vi "Tool Common analog Variables.vi"(11 "error in (no error)":errorcluster, 13 "Tool folder name":string) -> (8 "Common Variables Fixed":T7[](array[typedef]) {"Default Scaling"."Offset" format="%.5f"; "Default Scaling"."Gain" format="%.5f"}, 10 "Common variables User settigns":T1[](array[typedef]) {"Scaling"."Offset" format="%.5f"; "Scaling"."Gain" format="%.5f"; "Limits and responces"."Limits"."H" format="%.3f"; "Limits and responces"."Limits"."L" format="%.3f"; "Limits and responces"."Limits"."HH" format="%.3f"; "Limits and responces"."Limits"."LL" format="%.3f"; "Limits and responces"."HH"."Action" items=["No Action", "Turn Off HV"]; "Limits and responces"."H"."Action" items=["No Action", "Turn Off HV"]; "Limits and responces"."L"."Action" items=["No Action", "Turn Off HV"]; "Limits and responces"."LL"."Action" items=["No Action", "Turn Off HV"]; "Limits and responces"."Technical Error(NA)"."Action" items=["No Action", "Turn Off HV"]}, 15 "error out":errorcluster)   [LabVIEW 2011]
uses:
  Measurments Handling/Fixed Analog Channel Definition.ctl
  Measurments Handling/Update frequensies.ctl
  Measurments Handling/Channel catagory Enum.ctl
  Measurments Handling/Scaling.ctl
  Measurments Handling/User Setting Analog Channel Bg.ctl
  Measurments Handling/Alarm Setup Analog.ctl
  Measurments Handling/Alarm Responce.ctl
  Measurments Handling/Action List.ctl
  Measurments Handling/Limits.ctl
  Tool/Stroker/High level/Variable List Stroker Analog.ctl
  <vilib>/Utility/VariantDataType/GetNumericInfo.vi
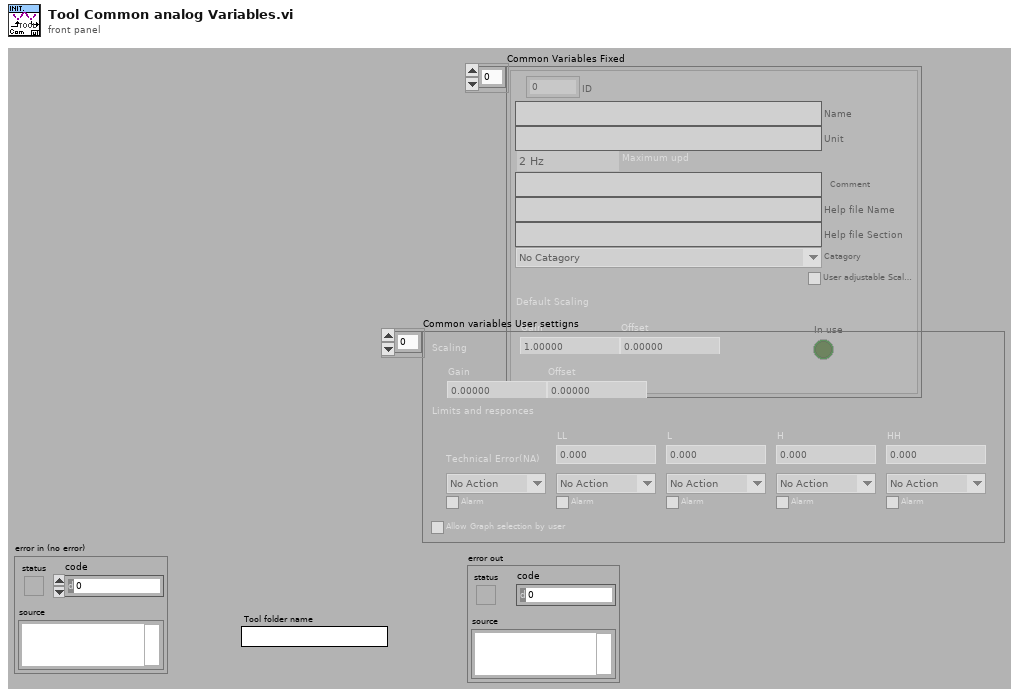
[diagram p1: front panel]
types:
  T1 = typedef "User Setting Analog Channel Bg.ctl" = cluster{"Scaling":T2, "Limits and responces":T3, "Allow Graph selection by user":bool}
  T2 = typedef "Scaling.ctl" = cluster{"Gain":dbl, "Offset":dbl}
  T3 = typedef "Alarm Setup Analog.ctl" = cluster{"Technical Error(NA)":T4, "LL":T4, "L":T4, "H":T4, "HH":T4, "Limits":T6}
  T4 = typedef "Alarm Responce.ctl" = cluster{"Action":T5, "Alarm":bool}
  T5 = typedef "Action List.ctl" = u16
  T6 = typedef "Limits.ctl" = cluster{"LL":dbl, "L":dbl, "H":dbl, "HH":dbl}
  T7 = typedef "Fixed Analog Channel Definition.ctl" = cluster{"ID":u16, "Name":string, "Unit":string, "Maximum upd":T8, "Comment":string, "Help file Name":string, "Help file Section ":string, "Catagory":T9, "User adjustable Scaling":bool, "Default Scaling":T2, "In use":bool}
  T8 = typedef "Update frequensies.ctl" = enum16{"2 Hz", "1 Hz", "0.1 Hz"}
  T9 = typedef "Channel catagory Enum.ctl" = enum16{"No Catagory", "Power", "Temperature", "Pressure"}
  T10 = typedef "Variable List Stroker Analog.ctl" = enum16{"Tool max Temperature", "Solenoid Temp", "Tool supply Voltage", "Tool (Controller) Current", "Tool Acceleration X", "Tool Acceleration Y", "Tool Acceleration Z", "Controller Temp", "Tool Acceleration Sum", "Tool Inclination", "Tool Rotation", "Tool Stroke Extension", "Tool GP Sensor 1", "Tool GP Sensor 2", "Tool (Pressure 1) Temp", "Tool Pressure 1", "Tool (Pressure 2) Temp", "Tool Pressure 2", "Do not use (SIF)", "Do not use (SOF)", "Stroke Force", "PSU Temp", "Head Voltage", "PSU Main Voltage out", "PSU Main Current out", "Tension Sub1 Temp", "Tool Tension Sub1", "Tension Sub2 Temp", "Tool Tension Sub2"}
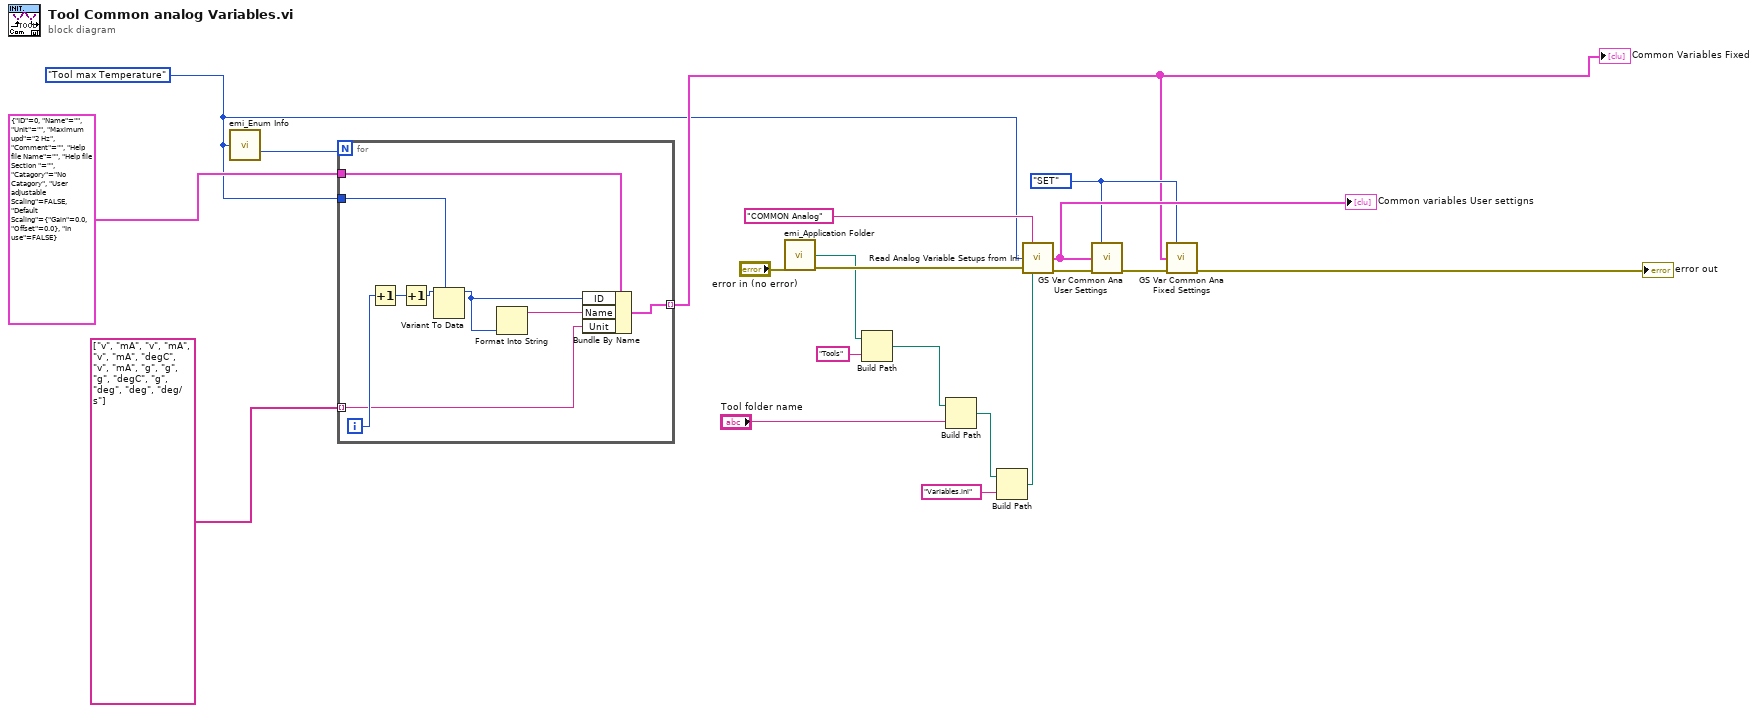
[diagram p0: block diagram]
diagram:
  w7 = Variable_List_Stroker_Analog."Tool max Temperature" ("Action")
  w15 = enum16{"GET", "SET"}."SET" ("Action(GET)")
  n1 = call "emi_Enum Info.vi"("Enum"=w7) -> ("Numb Elements"=w6:i32)  [unwired: 11 in, 3 out]
  n2 = for {
    N: w6 -> [_]
    tunnel: w7 -> [w27]
    tunnel: T7 {"ID"=0, "Name"="", "Unit"="", "Maximum upd"=enum."2 Hz", "Comment"="", "Help file Name"="", "Help file Section "="", "Catagory"=enum."No Catagory", "User adjustable Scaling"=FALSE, "Default Scaling"={"Gain"=0.0, "Offset"=0.0}, "In use"=FALSE} ("Variable Defenition") -> [w22]
    tunnel: [w23] -> w8 mode=indexing
    tunnel: string[] ["v", "mA", "v", "mA", "v", "mA", "degC", "v", "mA", "g", "g", "g", "degC", "g", "deg", "deg", "deg/s"] -> [w21] mode=indexing
    i -> [w29]
    n3 = Increment(x=w29) -> (x+1=w28:i32)
    n4 = Increment(x=w28) -> (x+1=w26:i32)
    n5 = Variant To Data(type=w27, Variant=w26) -> (data=w24:T10)  [unwired: 1 in, 1 out]
    n6 = Format Into String(w24) -> (resulting string=w25:string)  [unwired: 3 in, 1 out]
    n7 = Bundle By Name(cluster=w22, "ID"=w24, "Name"=w25, "Unit"=w21) -> (w23:T7)
  }
  "Common Variables Fixed" <- w8
  n8 = call "emi_Application Folder.vi"("error in (no error)"="error in (no error)") -> ("Dir"=w2:path, "error out"=w11:errorcluster)  [unwired: 13 in]
  n9 = Build Path(base path=w2, name or relative path="Tools") -> (appended path=w1:path)
  n10 = Build Path(base path=w1, name or relative path="Tool folder name") -> (appended path=w4:path)
  n11 = Build Path(base path=w4, name or relative path="Variables.ini") -> (appended path=w10:path)
  n12 = call "Read Analog Variable Setups from Ini.vi"("error in (no error)"=w11, "Path"=w10, "Enum with Variable List"=w7, "Section(\"Default\")"="COMMON Analog" ("Section(\"Default\")")) -> ("error out"=w19:errorcluster, "Analog User settigns"=w18:T1[])  [unwired: 10 in]
  "Common variables User settigns" <- w18
  n13 = call "GS Var Common Ana User Settings.vi"("Action(GET)"=w15, "Common variables User settigns in"=w18, "error in (no error)"=w19) -> ("error out"=w17:errorcluster)  [unwired: 10 in, 2 out]
  n14 = call "GS Var Common Ana Fixed Settings.vi"("Action(GET)"=w15, "Common AAnalog Var Fixed in"=w8, "error in (no error)"=w17) -> ("error out"=→"error out":errorcluster)  [unwired: 10 in, 2 out]
